vi "Display PDF File for Preview.vi"(8 "Data Directories":string[](array[string]), 11 "PDF file":path) -> (0 "error out":errorcluster, 3 "Filename Out":string)   [LabVIEW 2021]
doc: "Use this VI to display a PDF document in a dialog box."
uses:
  Globals/Constants_global.vi
panel:
  out "Files already created":string[](array[string])
  in  "Filename":string(combo)
  in  "Save":bool
  in  "Don't Save this Plot":bool
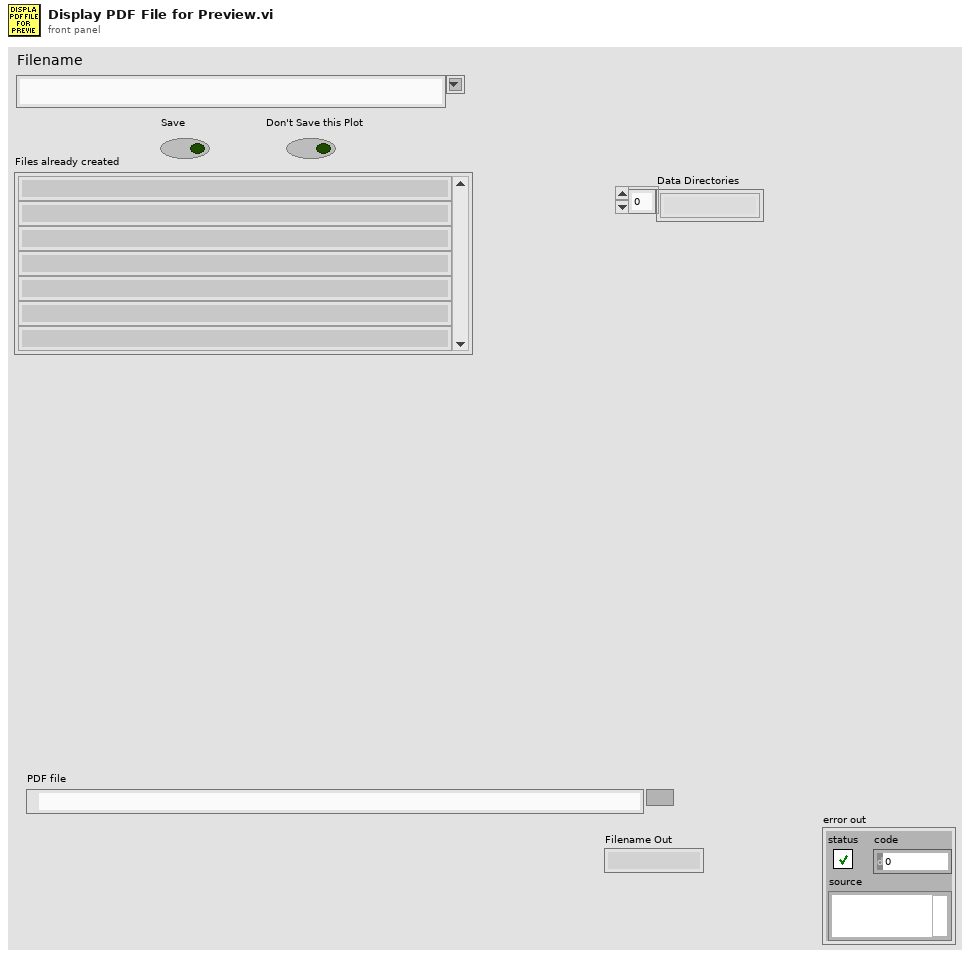
[diagram p1: front panel]
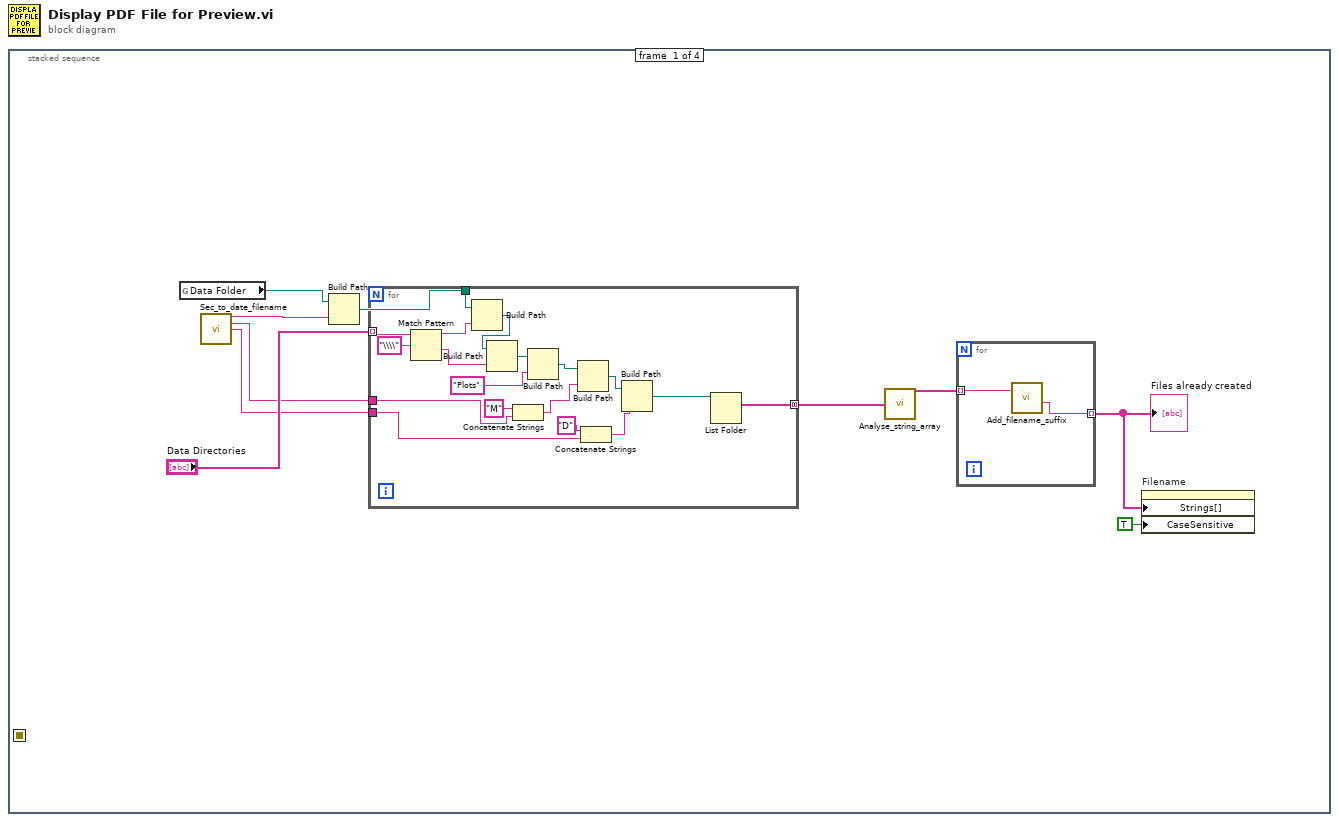
[diagram p0: block diagram]
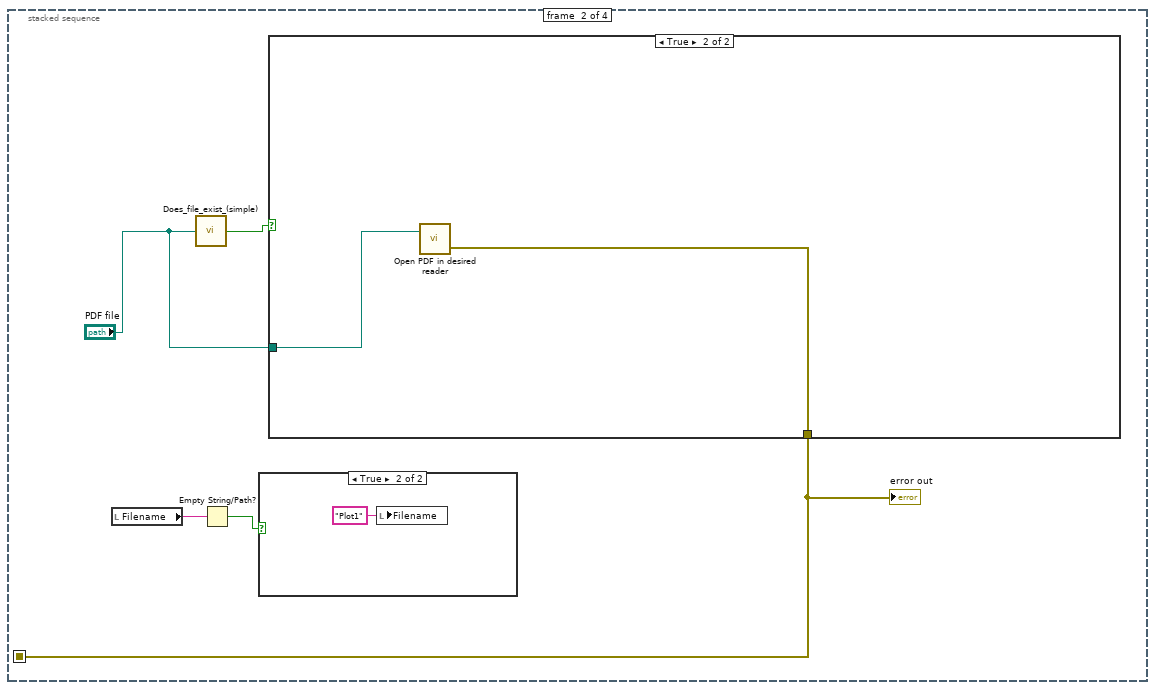
[diagram p2: hidden frame]
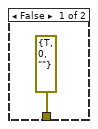
[diagram p4: hidden frame]
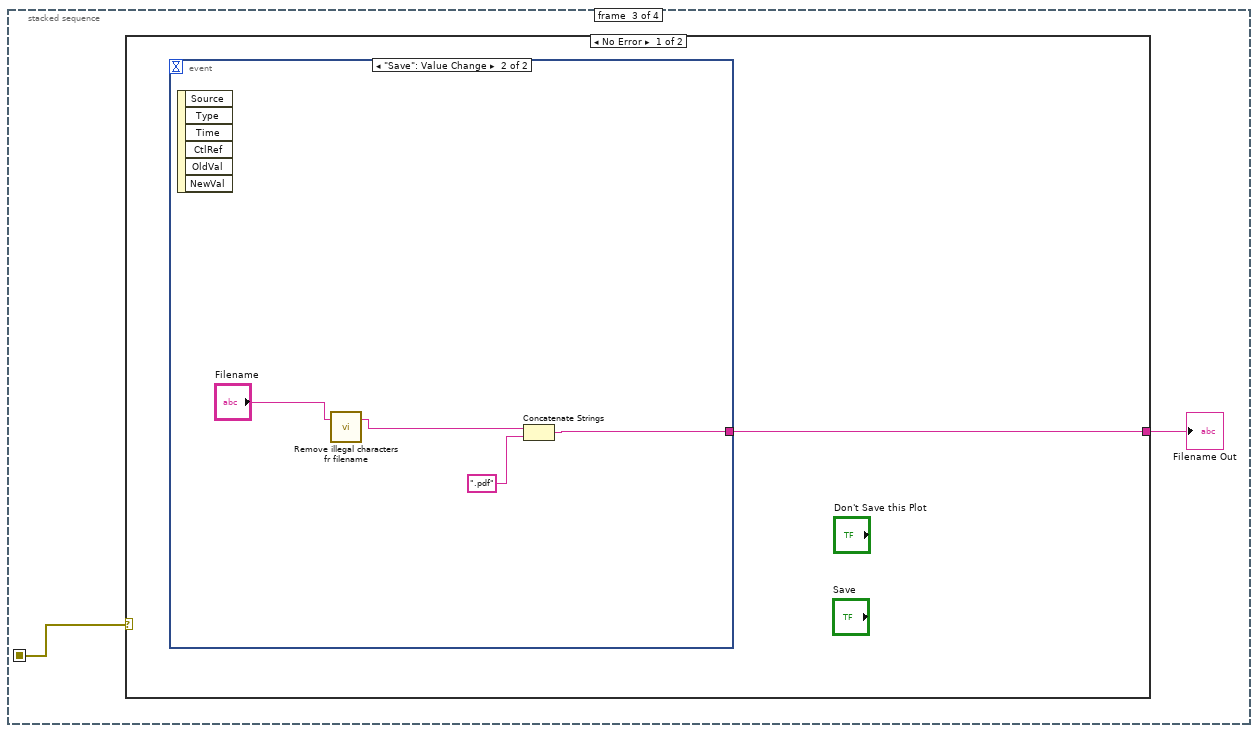
[diagram p5: hidden frame]
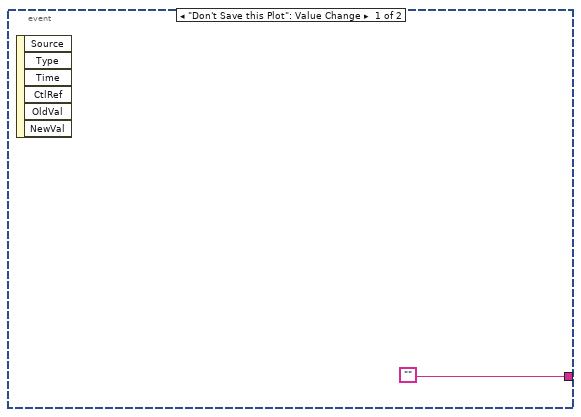
[diagram p6: hidden frame]
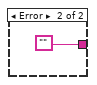
[diagram p7: hidden frame]
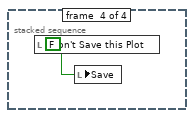
[diagram p8: hidden frame]
diagram:
  n1 = stacked-sequence {
    seq-local: [_ w35 _ _] -> [_ _ w41 _]
    frame #0 {
      n2 = global read "Constants_global.vi" "Data Folder"() -> (w8:path)
      n3 = call "Sec_to_date_filename.vi"() -> ("YYYY"=w7:string, "mm-YYYY"=w3:string, "DD"=w2:string)  [unwired: 6 in, 7 out]
      n4 = Build Path(base path=w8, name or relative path=w7) -> (appended path=w9:path)
      n5 = for {
        tunnel: "Data Directories" -> [w30] mode=indexing
        tunnel: w9 -> [w28]
        tunnel: w3 -> [w19]
        tunnel: w2 -> [w16]
        tunnel: [w13] -> w6 mode=concatenating
        n6 = Match Pattern(string=w30, regular expression="\\\\") -> (before substring=w26:string, after substring=w25:string)  [unwired: 1 in, 2 out]
        n7 = Build Path(base path=w28, name or relative path=w26) -> (appended path=w27:path)
        n8 = Build Path(base path=w27, name or relative path=w25) -> (appended path=w24:path)
        n9 = Concatenate Strings("M" ("string"), w19) -> (w21:string)
        n10 = Build Path(base path=w24, name or relative path="Plots") -> (appended path=w22:path)
        n11 = Build Path(base path=w22, name or relative path=w21) -> (appended path=w18:path)
        n12 = Concatenate Strings("D" ("string"), w16) -> (w15:string)
        n13 = Build Path(base path=w18, name or relative path=w15) -> (appended path=w14:path)
        n14 = List Folder(path=w14) -> (filenames=w13:string[])  [unwired: 3 in, 3 out]
      }
      n15 = call "Analyse_string_array.vi"("String array"=w6) -> ("Unique strings"=w5:string[])  [unwired: 1 in, 1 out]
      n16 = for {
        tunnel: w5 -> [w12] mode=indexing
        tunnel: [w11] -> w4 mode=indexing
        n17 = call "Add_filename_suffix.vi"("Filename"=w12) -> ("Base name"=w11:string)  [unwired: 1 in, 3 out]
      }
      "Files already created" <- w4
      n18 = property on="Filename" class="CmbBox"("Strings[]"=w4, "CaseSensitive"=TRUE ("Case Sensitive Pop-up")) -> ()  [unwired: 2 in, 2 out]
    }
    frame #1 {
      n19 = local read "Filename"() -> (w33:string)
      n20 = call "Does_file_exist_(simple).vi"("Pathname"="PDF file") -> ("exists?"=w34:bool)
      n21 = Empty String/Path?(string/path=w33) -> (empty?=w32:bool)
      n22 = case shown="True" w32 {
        frame False {
        }
        frame True {
          n23 = local write "Filename"("Plot1" ("Filename")) -> ()
        }
      }
      n24 = case shown="True" w34 {
        tunnel: [errorcluster {"status"=TRUE, "code"=0, "source"=""} ("error out") w38] -> w35
        tunnel: "PDF file" -> [_ w39]
        frame False {
        }
        frame True {
          n25 = call "Open PDF in desired reader.vi"("Path"=w39) -> ("error out"=w38:errorcluster)  [unwired: 2 in]
        }
      }
      "error out" <- w35
    }
    frame #2 {
      n26 = case shown="No Error" w41 {
        tunnel: [w42 ""] -> w40
        frame No Error {
          n27 = event shown="[1] \"Save\": Value Change" {
            selector: _ -> [_ _]
            dyn-events: _ -> [_ _]
            timeout: _ -> [_ _]
            tunnel: ["" w46] -> w42
            event "Don't Save this Plot": Value Change {
              n28 = event-data() -> ()  [unwired: 1 in, 6 out]
            }
            event "Save": Value Change {
              n29 = event-data() -> ()  [unwired: 1 in, 6 out]
              n30 = call "Remove illegal characters fr filename.vi"("Filename In"="Filename") -> ("Cleaned Filename"=w44:string)  [unwired: 2 in]
              n31 = Concatenate Strings(w44, ".pdf" ("string")) -> (w46:string)
            }
          }
        }
        frame Error {
        }
      }
      "Filename Out" <- w40
    }
    frame #3 {
      w49 = FALSE ("Delete")
      n32 = local write "Don't Save this Plot"(w49) -> ()
      n33 = local write "Save"(w49) -> ()
    }
  }
